vi "determineslope.vi"() -> ()   [LabVIEW 2010]
uses:
  <vilib>/Analysis/NI_AALPro.lvlib
panel:
  out "slope":dbl format="%.7f"
  out "error out 2":errorcluster
  out "XY Graph":cluster{dbl[], dbl[]}(graph)
  in  "Wait/s":dbl format="%.2f"
  in  "Step":dbl format="%.2f"
  in  "error in (no error)":errorcluster
  in  "Stop":dbl format="%.2f"
  in  "Start":dbl format="%.2f"
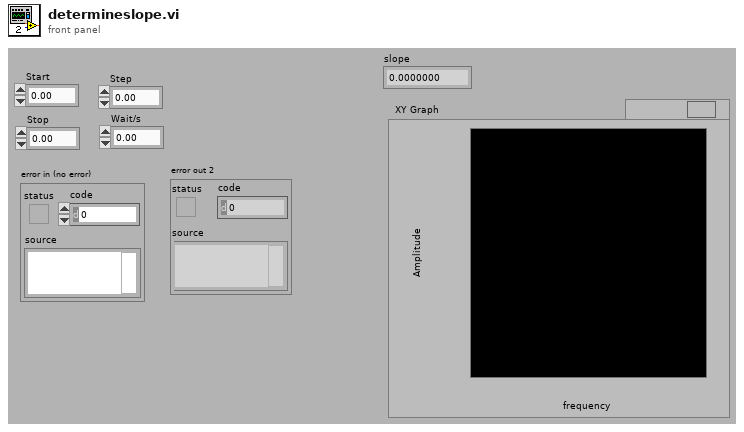
[diagram p1: front panel]
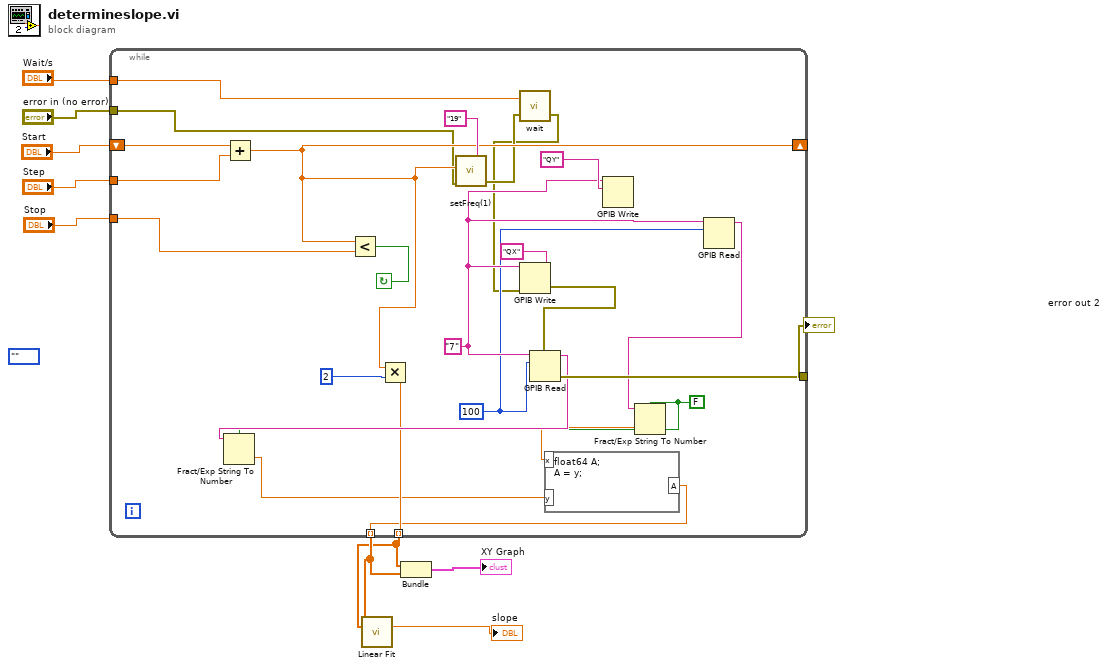
[diagram p0: block diagram]
diagram:
  (unwired) enum16{""}.""
  n1 = while {
    tunnel: "error in (no error)" -> [w13]
    shift-right: [w14] -> _
    shift-left: "Start" -> [w32]
    tunnel: "Step" -> [w34]
    tunnel: "Stop" -> [w33]
    tunnel: "Wait/s" -> [w30]
    tunnel: [w28] -> w5
    tunnel: [w17] -> w3 mode=indexing
    tunnel: [w23] -> w2 mode=indexing
    stop <- w31 continue-if-true
    w16 = FALSE
    w15 = 100
    w21 = "7"
    n2 = Add(x=w32, y=w34) -> (x+y=w14:dbl)
    n3 = Less?(x=w14, y=w33) -> (x < y?=w31:bool)
    n4 = Multiply(x=w14, y=2) -> (x*y=w23:dbl)
    n5 = call "setFreq(1).vi"("error in"=w13, "Frequenz in Hz"=w14, "address string"="19") -> ("error out"=w12:errorcluster)  [unwired: 3 in]
    n6 = call "wait.vi"("error in"=w12, "Wartezeit in Sek"=w30) -> ("error out"=w11:errorcluster)  [unwired: 1 in]
    n7 = GPIB Write(0:w21, 1:"QX", 3:w11) -> (6:w26:errorcluster)  [unwired: 2 in, 1 out]
    n8 = GPIB Read(0:w21, 1:w15, 3:w26) -> (5:w25:string, 7:w28:errorcluster)  [unwired: 2 in, 1 out]
    n9 = Fract/Exp String To Number(use system decimal point (T)=w16, string=w25) -> (number=w18:dbl)  [unwired: 2 in, 1 out]
    n10 = GPIB Write(0:w21, 1:"QY") -> ()  [unwired: 3 in, 2 out]
    n11 = GPIB Read(0:w21, 1:w15) -> (5:w20:string)  [unwired: 3 in, 2 out]
    n12 = Fract/Exp String To Number(use system decimal point (T)=w16, string=w20) -> (number=w19:dbl)  [unwired: 2 in, 1 out]
    n13 = formula code="float64 A;\nA = y;"("x"=w19, "y"=w18) -> ("A"=w17:dbl)
  }
  "error out 2" <- w5
  n14 = call <vilib>:"Linear Fit.vi"("Y"=w3, "X"=w2) -> ("slope"=→"slope":dbl)  [unwired: 9 in, 4 out]
  n15 = Bundle(w2, w3) -> (→"XY Graph":cluster{dbl[], dbl[]})  [unwired: 1 in]
